vi "Launch_Sequencer.vi"(8 "error in (no error)":errorcluster caption="entrée d'erreur (pas d'erreur)") -> (0 "error out":errorcluster caption="sortie d'erreur", 1 "Result":bool, 2 "Result Sequence":T3(array[cluster]), 3 "Json_String":string)   [LabVIEW 2020, in "Library Core.lvlib" / "Sequencer (Default).lvclass"]
uses:
  Sequencer (Default).lvclass
  Commun VI/TypeDef/Commande Test/Commande Value Type.ctl
  Commun VI/TypeDef/Commande Test/Commande Type Test.ctl
  Variable Test.vi
  Commun VI/Library Commun.lvlib
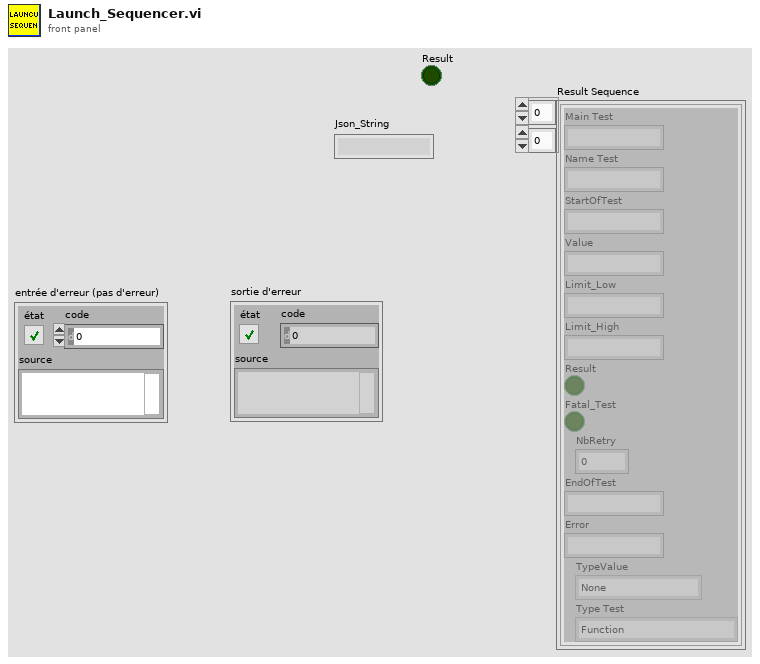
[diagram p1: front panel]
types:
  T1 = typedef "Library Commun.lvlib/Commande Value Type.ctl" = enum16{"None", "String", "Number", "Timestamp", "Boolean", "Array"}
  T2 = typedef "Library Commun.lvlib/Commande Type Test.ctl" = enum16{"Function", "Test", "Calculation"}
  T3 = cluster{"Main Test":string, "Name Test":string, "StartOfTest":string, "Value":string, "Limit_Low":string, "Limit_High":string, "Result":bool, "Fatal_Test":bool, "NbRetry":dbl, "EndOfTest":string, "Error":string, "TypeValue":T1, "Type Test":T2}[][]
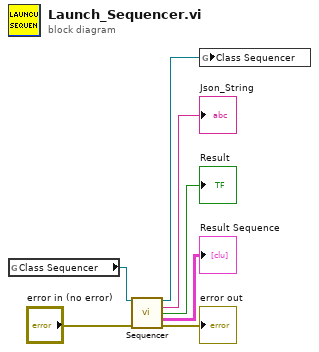
[diagram p0: block diagram]
diagram:
  n1 = global read "Variable Test.vi" "Class Sequencer"() -> (w4:refnum<class "Sequencer (Default).lvclass">)
  n2 = call-dynamic "Sequencer.vi"("Test (Default) en entrée"=w4, "error in (no error)"="error in (no error)") -> ("Test (Default) en sortie"=w3:refnum<class "Sequencer (Default).lvclass">, "Json_String"=→"Json_String":string, "Result"=→"Result":bool, "Result Sequence"=→"Result Sequence":T3, "error out"=→"error out":errorcluster)  [unwired: 9 in]
  n3 = global write "Variable Test.vi" "Class Sequencer"(w3) -> ()
